vi "PCO_Grab.vi"(8 "entrée d'erreur (pas d'erreur)":errorcluster, 9 "notifier out":refnum<notifier>, 10 "dwImgCount":u32=10 caption="Required Number of Images" max=2397, 11 "Camera en entrée":refnum<class "Camera.lvclass">) -> (0 "sortie d'erreur":errorcluster, 1 "meta_data_list":T1(array[cluster]), 2 "Raw data (U16)":u16[][][](array[numeric]), 3 "Camera en sortie":refnum<class "Camera.lvclass">)   [LabVIEW 2026]
uses:
  <instrlib>/PCO_SDK/File Group 0/vi.lib/Excelitas PCO GmbH/pco.labview/camera/Camera.lvclass
  <instrlib>/PCO_SDK/File Group 0/vi.lib/Excelitas PCO GmbH/pco.labview/pco.sdk/TimingControl/TimingControl.lvlib
panel:
  out "recorded_image_count":u32
  out "Recorded Images":u32=1
  out "Image(U16)":u16[][](graph)
  out "x = y ?":bool
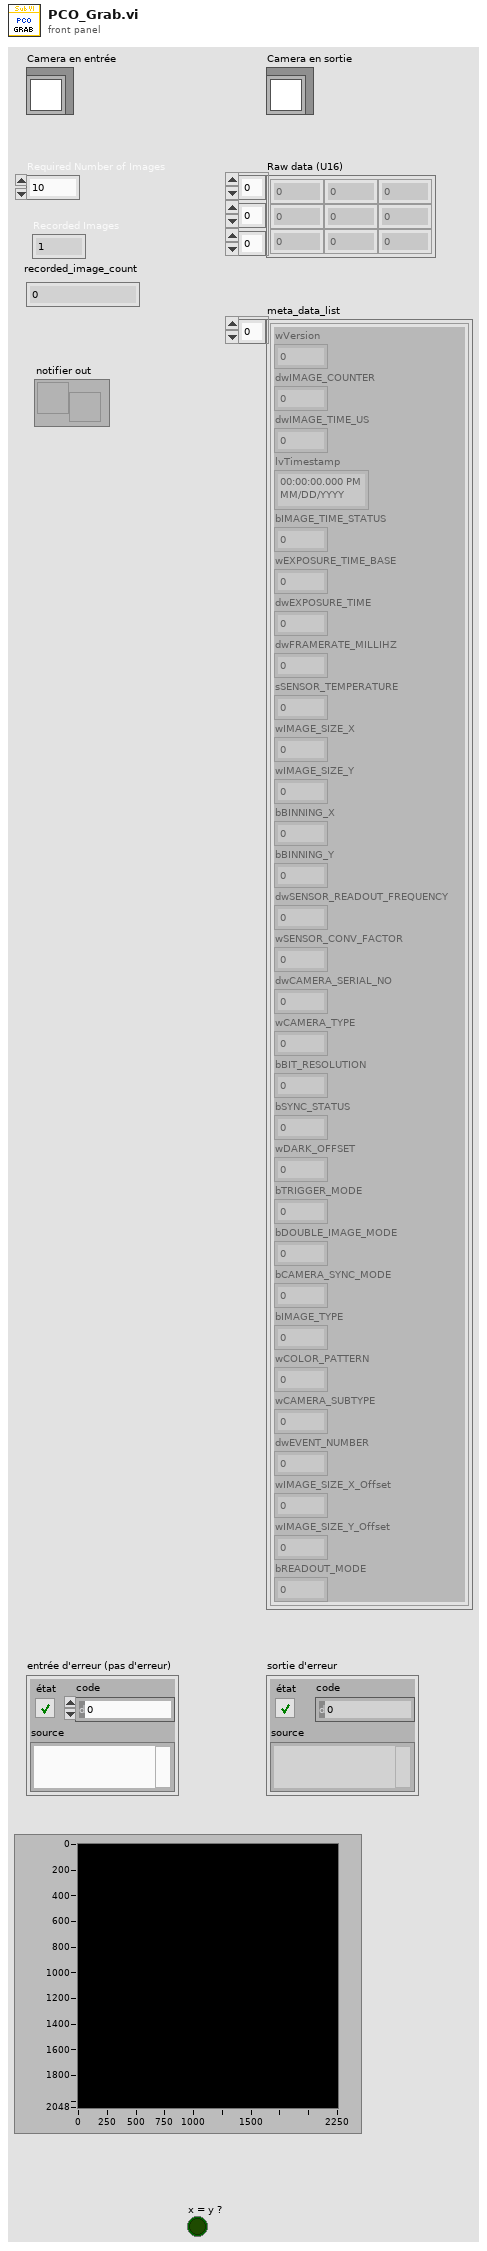
[diagram p1: front panel]
types:
  T1 = cluster{"wVersion":u16, "dwIMAGE_COUNTER":u32, "dwIMAGE_TIME_US":u32, "lvTimestamp":timestamp, "bIMAGE_TIME_STATUS":u8, "wEXPOSURE_TIME_BASE":u16, "dwEXPOSURE_TIME":u32, "dwFRAMERATE_MILLIHZ":u32, "sSENSOR_TEMPERATURE":i16, "wIMAGE_SIZE_X":u16, "wIMAGE_SIZE_Y":u16, "bBINNING_X":u8, "bBINNING_Y":u8, "dwSENSOR_READOUT_FREQUENCY":u32, "wSENSOR_CONV_FACTOR":u16, "dwCAMERA_SERIAL_NO":u32, "wCAMERA_TYPE":u16, "bBIT_RESOLUTION":u8, "bSYNC_STATUS":u8, "wDARK_OFFSET":u16, "bTRIGGER_MODE":u8, "bDOUBLE_IMAGE_MODE":u8, "bCAMERA_SYNC_MODE":u8, "bIMAGE_TYPE":u8, "wCOLOR_PATTERN":u16, "wCAMERA_SUBTYPE":u16, "dwEVENT_NUMBER":u32, "wIMAGE_SIZE_X_Offset":u16, "wIMAGE_SIZE_Y_Offset":u16, "bREADOUT_MODE":u8}[]
  T2 = enum16{"Undefined", "Mono8", "Mono16", "BGRA8", "RGBA8", "BGRA16", "RGBA16", "CompressedMono8"}
  T3 = enum16{"auto sequence", "software trigger", "external exposure start", "external exposure control"}
  T4 = enum16{"sequence", "sequence non blocking", "ring buffer", "fifo", "sequence_dpcore", "sequence_non_blocking_dpcore", "ring_buffer_dpcore", "fifo_dpcore", "tif", "multitif", "pcoraw", "b16", "dicom", "multidicom", "camram_ring", "camram_segment"}
  T5 = typedef "Camera.lvclass/binning.ctl" = cluster{"vert":u16, "horz":u16, "mode":u16}
  T6 = cluster{"exposure_time_s":dbl, "delay_time_s":dbl, "roi":cluster{"x0":u64, "y0":u64, "x1":u64, "y1":u64}, "timestamp_mode":u16, "pixelrate":u32, "trigger_mode":u16, "acquire_mode":u16, "metadata_mode":u16, "noisefilter_mode":u16, "pixel_format":u32, "binning":T5, "auto_exposure":cluster{"region":u16, "min_exposure_s":dbl, "max_exposure_s":dbl}}
  T7 = cluster{"wSignalNum":u16, "wEnabled":u16, "wType":u16, "wPolarity":u16, "wFilterSetting":u16, "wSelected":u16, "dwParameter":u32[], "dwSignalFunctionality":u32[]}
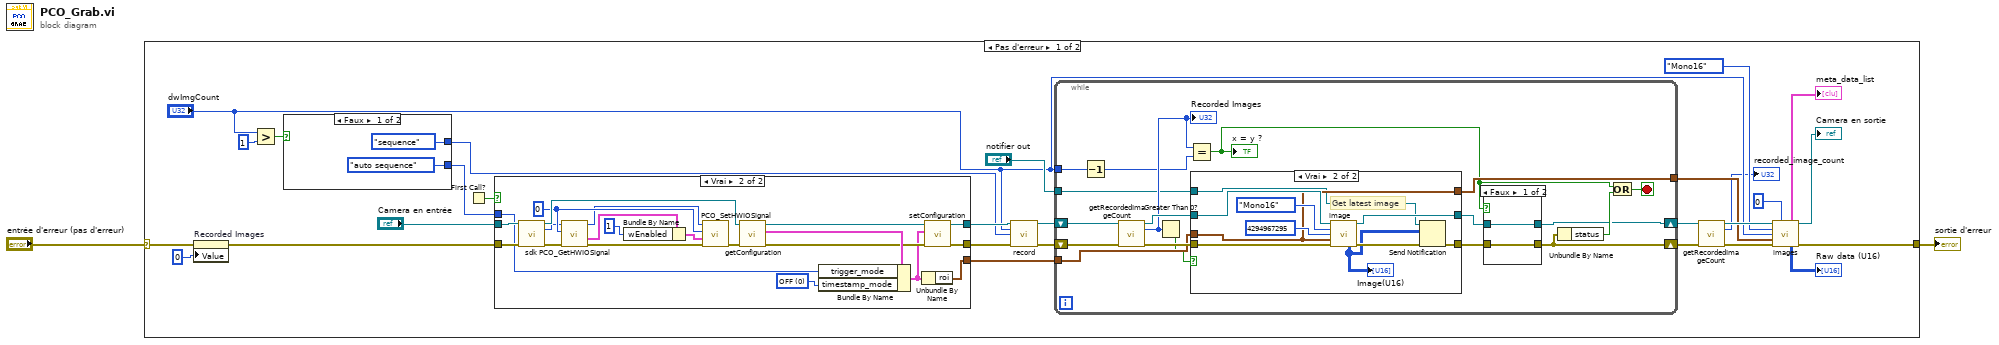
[diagram p0: block diagram]
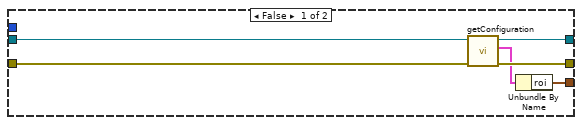
[diagram p2: hidden frame]
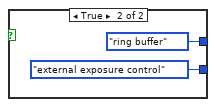
[diagram p3: hidden frame]
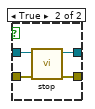
[diagram p5: hidden frame]
diagram:
  n1 = case shown="Pas d'erreur" "entrée d'erreur (pas d'erreur)" {
    selector: "entrée d'erreur (pas d'erreur)" -> [w20 w99]
    tunnel: [w16 w99] -> w2
    frame No Error {
      n2 = property on="Recorded Images" class="NumNb (strict)"(error in=w20, "Value"=u32 0 ("Recorded Images")) -> (error out=w19:errorcluster)  [unwired: 1 in, 1 out]
      n3 = Greater?(x="dwImgCount", y=u32 1 ("x")) -> (0:w8:bool)
      n4 = case shown="Faux" w8 {
        tunnel: [T4."sequence" ("record_mode") T4."ring buffer" ("record_mode")] -> w9
        tunnel: [T3."auto sequence" ("TriggerMode") T3."external exposure control" ("TriggerMode")] -> w5
        frame False {
        }
        frame True {
        }
      }
      n5 = First Call?() -> (First Call?: T/F=w3:bool)
      n6 = case shown="Vrai" w3 {
        tunnel: [w33 w57] -> w30
        tunnel: [w34 w56] -> w29
        tunnel: "Camera en entrée" -> [w36 w42]
        tunnel: [w31 w39] -> w23
        tunnel: w19 -> [w35 w38]
        tunnel: w5 -> [_ w37]
        frame False {
          n7 = call-dynamic "getConfiguration.vi"("error in (no error)"=w35, "Camera in"=w36) -> ("error out"=w34:errorcluster, "configuration"=w32:T6, "Camera out"=w33:refnum<class "Camera.lvclass">)  [unwired: 7 in]
          n8 = Unbundle By Name(w32) -> ("roi"=w31:cluster{"x0":u64, "y0":u64, "x1":u64, "y1":u64})
        }
        frame True {
          w45 = u16 0 items=["OFF", "Binary", "Binary+ASCII", "ASCII"] ("wTimeStampMode")
          w51 = u16 0 ("wSignalNum")
          n9 = call-dynamic "sdk.vi"("Camera in"=w42, "error in (no error)"=w38) -> ("Camera out"=w55:refnum<class "Camera.lvclass">, "sdk"=w47:u64, "error out"=w54:errorcluster)  [unwired: 11 in]
          n10 = call <instrlib>:"PCO_GetHWIOSignal.vi"("error in (no error)"=w54, "wSignalNum"=w51, "ph"=w47) -> ("error out"=w49:errorcluster, "strSignal"=w53:T7, "ph out"=w48:u64)  [unwired: 5 in, 1 out]
          n11 = Bundle By Name(cluster=w53, "wEnabled"=u16 1) -> (w50:T7)
          n12 = call <instrlib>:"PCO_SetHWIOSignal.vi"("error in (no error)"=w49, "strSignal"=w50, "wSignalNum"=w51, "ph"=w48) -> ("error out"=w41:errorcluster)  [unwired: 5 in, 2 out]
          n13 = call-dynamic "getConfiguration.vi"("error in (no error)"=w41, "Camera in"=w55) -> ("error out"=w43:errorcluster, "configuration"=w46:T6, "Camera out"=w44:refnum<class "Camera.lvclass">)  [unwired: 7 in]
          n14 = Bundle By Name(cluster=w46, "trigger_mode"=w37, "timestamp_mode"=w45) -> (w40:T6)
          n15 = Unbundle By Name(w40) -> ("roi"=w39:cluster{"x0":u64, "y0":u64, "x1":u64, "y1":u64})
          n16 = call-dynamic "setConfiguration.vi"("error in (no error)"=w43, "configuration"=w40, "Camera in"=w44) -> ("error out"=w56:errorcluster, "Camera out"=w57:refnum<class "Camera.lvclass">)  [unwired: 7 in]
        }
      }
      n17 = call-dynamic "record.vi"("Camera in"=w30, "num_images"="dwImgCount", "record_mode"=w9, "error in (no error)"=w29) -> ("Camera out"=w26:refnum<class "Camera.lvclass">, "error out"=w25:errorcluster)  [unwired: 10 in]
      n18 = while {
        shift-right: [w72] -> w28
        shift-left: w25 -> [w62]
        shift-right: [w73] -> w27
        shift-left: w26 -> [w63]
        tunnel: "dwImgCount" -> [w70]
        tunnel: w23 -> [w69]
        tunnel: [w68] -> w12
        tunnel: "notifier out" -> [w67]
        stop <- w79 stop-if-true
        n19 = Decrement(x=w70) -> (x-1=w65:u32)
        n20 = call-dynamic "getRecordedImageCount.vi"("Camera in"=w63, "error in (no error)"=w62) -> ("Camera out"=w75:refnum<class "Camera.lvclass">, "recorded_image_count"=w71:u32, "error out"=w76:errorcluster)  [unwired: 11 in]
        "Recorded Images" <- w71
        n21 = Greater Than 0?(x=w71) -> (x > 0?=w64:bool)
        n22 = Equal?(x=w71, y=w65) -> (x = y?=w66:bool)
        "x = y ?" <- w66
        n23 = case shown="Vrai" w64 {
          tunnel: [w81 w84] -> w77
          tunnel: w76 -> [w81 w91]
          tunnel: w75 -> [w82 w90]
          tunnel: [w82 w89] -> w74
          tunnel: w69 -> [w80 w87]
          tunnel: [w80 w87] -> w68
          tunnel: w67 -> [_ w86]
          frame False {
          }
          frame True {
            # "Get latest image"
            n24 = call-dynamic "image.vi"("Camera in"=w90, "data_format"=T2."Mono16", "image_index"=u32 4294967295 ("dwImgIdx"), "roi"=w87, "error in (no error)"=w91) -> ("Camera out"=w89:refnum<class "Camera.lvclass">, "raw_image (U16)"=w83:u16[][], "error out"=w85:errorcluster)  [unwired: 2 in, 6 out]
            "Image(U16)" <- w83
            n25 = Send Notification(notification=w83, notifier=w86, error in (no error)=w85) -> (error out=w84:errorcluster)  [unwired: 1 out]
          }
        }
        n26 = case shown="Faux" w66 {
          tunnel: w77 -> [w94 w95]
          tunnel: [w93 w97] -> w73
          tunnel: [w94 w98] -> w72
          tunnel: w74 -> [w93 w96]
          frame False {
          }
          frame True {
            n27 = call-dynamic "stop.vi"("error in (no error)"=w95, "Camera in"=w96) -> ("error out"=w98:errorcluster, "Camera out"=w97:refnum<class "Camera.lvclass">)  [unwired: 8 in]
          }
        }
        n28 = Unbundle By Name(w72) -> ("status"=w78:bool)
        n29 = Or(x=w66, y=w78) -> (x .or. y?=w79:bool)
      }
      n30 = call-dynamic "getRecordedImageCount.vi"("Camera in"=w27, "error in (no error)"=w28) -> ("Camera out"=w14:refnum<class "Camera.lvclass">, "recorded_image_count"=→"recorded_image_count":u32, "error out"=w17:errorcluster)  [unwired: 11 in]
      n31 = call-dynamic "images.vi"("Camera in"=w14, "start_index"=u32 0, "data_format"=T2."Mono16", "image_count"="dwImgCount", "roi"=w12, "error in (no error)"=w17) -> ("meta_data_list"=→"meta_data_list":T1, "Camera out"=→"Camera en sortie":refnum<class "Camera.lvclass">, "raw_image_list (U16)"=→"Raw data (U16)":u16[][][], "error out"=w16:errorcluster)  [unwired: 1 in, 5 out]
    }
    frame Error {
    }
  }
  "sortie d'erreur" <- w2
